vi "lua_gettop.vi"(8 "error in (no error)":errorcluster, 11 "lua_state_p":u64) -> (0 "error out":errorcluster, 2 "index":i32, 3 "lua_state_p out":u64)   [LabVIEW 2020, in "lua.dll.lvlib"]
uses:
  lua.dll.lvlib
  lua54.dll
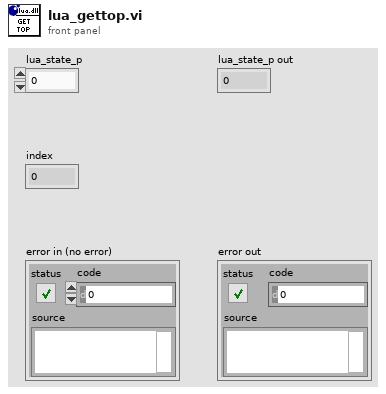
[diagram p1: front panel]
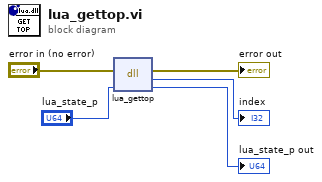
[diagram p0: block diagram]
diagram:
  n1 = dll-call lib="C:/Users/Nicholas Folse/Documents/workspace/github-tauterra.llc/Lua for LabVIEW/lib/lua.dll/lua54**.*" fn="lua_gettop"(error in="error in (no error)", "lua_state_p"="lua_state_p") -> (error out=→"error out":errorcluster, "return"=→"index":i32, "lua_state_p"=→"lua_state_p out":u64)  [unwired: 2 in, 1 out]
